vi "Autorun Generate JSON Request.vi"   [LabVIEW 2014, in "i3-docs.lvlib"]
uses:
  i3-docs.lvlib
  Generate JSON Report.vi
types:
  T1 = enum32{"Invalid", "Standard", "Closed", "Hidden", "Minimized", "Maximized"}
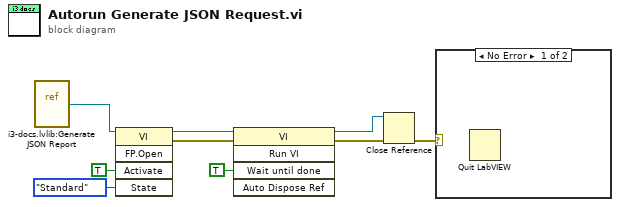
[diagram p0: block diagram]
diagram:
  n1 = vi-ref "i3-docs.lvlib:Generate JSON Report.vi"() -> (w1:refnum<vi>)
  n2 = invoke class="VI" method="FP.Open"(reference=w1, "Activate"=TRUE ("Activate?"), "State"=T1."Standard") -> (reference out=w4:refnum<vi>, error out=w5:errorcluster)  [unwired: 2 in, 3 out]
  n3 = invoke class="VI" method="Run VI"(reference=w4, error in=w5, "Wait until done"=TRUE ("Wait Until Done")) -> (reference out=w8:refnum<vi>, error out=w7:errorcluster)  [unwired: 2 in, 3 out]
  n4 = Close Reference(reference=w8, error in (no error)=w7) -> (error out=w6:errorcluster)
  n5 = case shown="No Error" w6 {
    frame No Error {
      n6 = Quit LabVIEW() -> ()  [unwired: 1 in]
    }
    frame Error {
    }
  }
